vi "Merge Default and Override-Example.vi"() -> ()   [LabVIEW 2015]
uses:
  <vilib>/addons/_JKI.lib/Serialization/JSON/JKI JSON Serialization.lvlib
panel:
  in  "Override":string="{\n  \"Name\": \"A\",\n  \"Dept\": \"Alpha\",\n  \"Array\": [\n    1,\n    2,\n    4\n  ],\n  \"ArrayOfClusters\": [\n    {\n      \"Name\": \"A1\",\n      \"Dept\": \"Alpha2\"\n    },\n    {\n      \"Name\": \"B1\",\n      \"Dept\": \"Beta1\"\n    }\n  ]\n}"
  in  "Default":string="{\n  \"Name\": \"A\",\n  \"Array\": [\n    1,\n    2,\n    3\n  ],\n  \"ArrayOfClusters\": [\n    {\n      \"Name\": \"A1\",\n      \"Dept\": \"Alpha1\"\n    },\n    {\n      \"Name\": \"A2\",\n      \"Dept\": \"Alpha2\"\n    },\n    {\n      \"Name\": \"B2\",\n      \"Dept\": \"Beta2\"\n    }\n  ]\n}"
  out "error out":errorcluster
  in  "error in":errorcluster
  out "JSON String out":string
  in  "Default":path=path "E:/JSON File Handling/Path to VCluster (Default and Override)/Report/Default JSON ZenGage Test.txt"
  in  "Override":path=path "E:/JSON File Handling/Path to VCluster (Default and Override)/Report/Override JSON ZenGage Test.txt"
  in  "Override":string
  in  "Default":string
  # "{\n  \"Name\": \"A\",\n  \"Array\": [\n    1,\n    2,\n    3\n  ],\n  \"ArrayOfClusters\": [\n    {\n      \"Name\": \"A1\",\n      \"Dept\": \"Alpha1\"\n    },\n    {\n      \"Name\": \"A2\",\n      \"Dept\": \"Alpha2\"\n    },\n    {\n      \"Name\": \"B2\",\n      \"Dept\": \"Beta2\"\n    }\n  ]\n}"
  # "{\n  \"Name\": \"A\",\n  \"Dept\": \"Alpha\",\n  \"Array\": [\n    1,\n    2,\n    4\n  ],\n  \"ArrayOfClusters\": [\n    {\n      \"Name\": \"A1\",\n      \"Dept\": \"Alpha2\"\n    },\n    {\n      \"Name\": \"B1\",\n      \"Dept\": \"Beta1\"\n    }\n  ]\n}"
  # "Press Ctrl+R to run the current \nprogram.\nThe following can be changed based\nupon the requirement :\n1. JSON String\n2. PathList (To Query the data)\n3. Data in\n4. Data out"
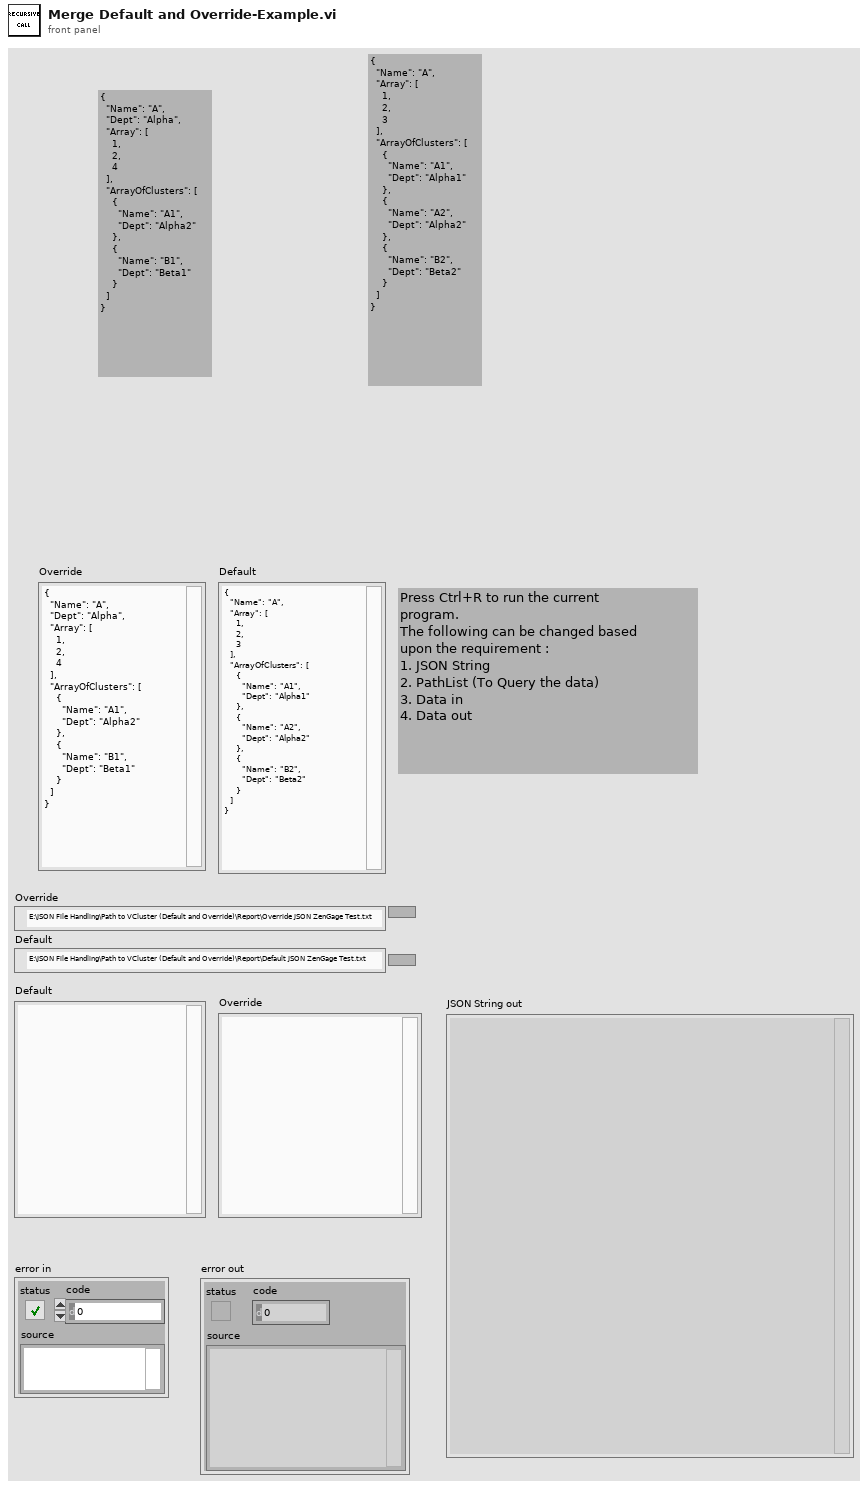
[diagram p1: front panel]
types:
  T1 = enum16{"open", "replace", "create", "open or create", "replace or create", "replace or create with confirmation"}
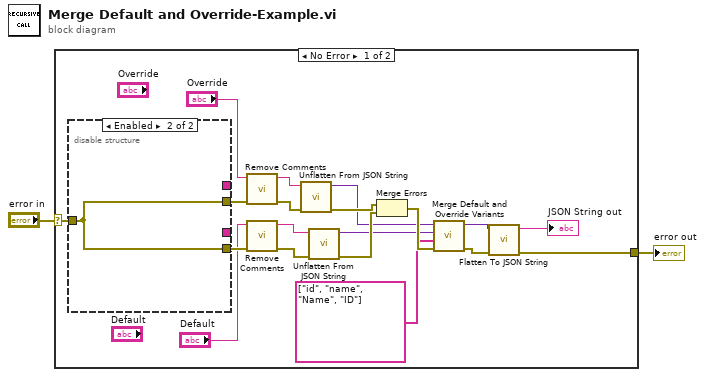
[diagram p0: block diagram]
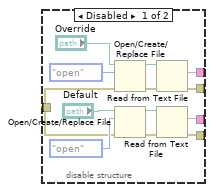
[diagram p2: hidden frame]
diagram:
  n1 = case shown="No Error" "error in" {
    selector: "error in" -> [w14 w36]
    tunnel: [w16 w36] -> w2
    frame No Error {
      n2 = disable-structure shown="Enabled" {
        disable-tunnel: w14 -> [w26 w35]
        disable-tunnel: [w25 w35] -> w11
        disable-tunnel: [w24 _] -> _
        disable-tunnel: [w23 _] -> _
        disable-tunnel: [w22 w35] -> w9
        frame Disabled {
          n3 = Open/Create/Replace File(file path (use dialog)="Override", error in=w26, operation (0:open)=T1."open") -> (refnum out=w31:refnum<file>, error out=w28:errorcluster)  [unwired: 3 in, 1 out]
          n4 = Open/Create/Replace File(file path (use dialog)="Default", error in=w26, operation (0:open)=T1."open") -> (refnum out=w32:refnum<file>, error out=w27:errorcluster)  [unwired: 3 in, 1 out]
          n5 = Read from Text File(file (use dialog)=w31, error in=w28) -> (text=w23:string, error out=w22:errorcluster)  [unwired: 2 in, 2 out]
          n6 = Read from Text File(file (use dialog)=w32, error in=w27) -> (text=w24:string, error out=w25:errorcluster)  [unwired: 2 in, 2 out]
        }
        frame Enabled {
        }
      }
      n7 = call "Remove Comments.vi"("error in (no error)"=w9, "input string"="Override") -> ("error out"=w8:errorcluster, "output String"=w6:string)  [unwired: 7 in, 1 out]
      n8 = call "Remove Comments.vi"("error in (no error)"=w11, "input string"="Default") -> ("error out"=w10:errorcluster, "output String"=w7:string)  [unwired: 7 in, 1 out]
      n9 = call <vilib>:"Unflatten From JSON String.vi"("error in (no error)"=w8, "JSON String"=w6) -> ("error out"=w19:errorcluster, "Variant"=w15:variant)  [unwired: 8 in]
      n10 = call <vilib>:"Unflatten From JSON String.vi"("error in (no error)"=w10, "JSON String"=w7) -> ("error out"=w18:errorcluster, "Variant"=w12:variant)  [unwired: 8 in]
      n11 = Merge Errors(w19, w18) -> (w17:errorcluster)
      n12 = call "Merge Default and Override Variants.vi"("error in (no error)"=w17, "Array element check\nkeys"=string[] ["id", "name", "Name", "ID"] ("Array element check\nkeys"), "Default VCluster"=w12, "Override VCluster"=w15) -> ("error out"=w13:errorcluster, "Output Merged Cluster"=w20:variant)  [unwired: 6 in]
      n13 = call <vilib>:"Flatten To JSON String.vi"("error in (no error)"=w13, "Variant"=w20) -> ("error out"=w16:errorcluster, "JSON String"=→"JSON String out":string)  [unwired: 8 in]
    }
    frame Error {
    }
  }
  "error out" <- w2
